vi "Attributes_TCwfm.vi"(2 "data":waveform(dbl)[](array[waveform]), 3 "Refnum in":refnum<k21>) -> (0 "Array":waveform(dbl)[](array[waveform]), 1 "Refnum in 2":refnum<k21>)   [LabVIEW 2017]
uses:
  <resource>/objmgr/daqmx.rc
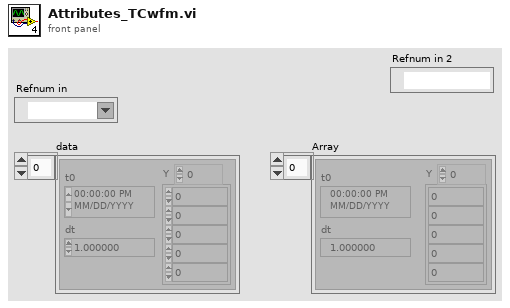
[diagram p1: front panel]
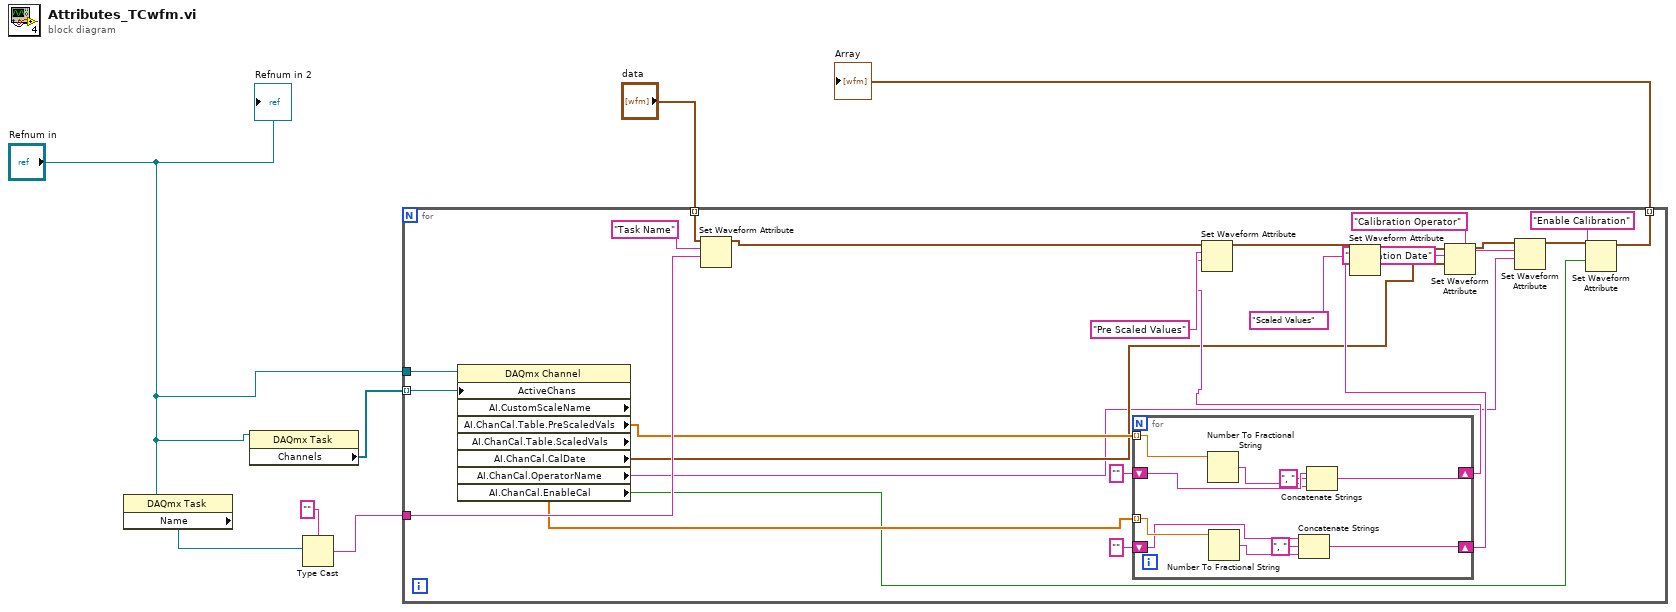
[diagram p0: block diagram]
diagram:
  n1 = property class="DAQmx Task"(reference="Refnum in") -> ("Name"=w4:refnum<k21>)  [unwired: 1 in, 2 out]
  n2 = property class="DAQmx Task"(reference="Refnum in") -> ("Channels"=w1:refnum<k21>[])  [unwired: 1 in, 2 out]
  n3 = Type Cast(type="", x=w4) -> (*(type *) &x=w6:string)
  n4 = for {
    tunnel: "data" -> [w31] mode=indexing
    tunnel: [w8] -> w7 mode=indexing
    tunnel: w6 -> [w30]
    tunnel: "Refnum in" -> [w28]
    tunnel: w1 -> [w27] mode=indexing
    n5 = property class="DAQmx Channel" props=["ActiveChans", "AI.CustomScaleName", "AI.ChanCal.Table.PreScaledVals", "AI.ChanCal.Table.ScaledVals", "AI.ChanCal.CalDate", "AI.ChanCal.OperatorName", "AI.ChanCal.EnableCal"](reference=w28, "ActiveChans"=w27) -> ("AI.ChanCal.Table.PreScaledVals"=w23:dbl[], "AI.ChanCal.Table.ScaledVals"=w22:dbl[], "AI.ChanCal.CalDate"=w16:timestamp, "AI.ChanCal.OperatorName"=w14:string, "AI.ChanCal.EnableCal"=w12:bool)  [unwired: 1 in, 3 out]
    n6 = Set Waveform Attribute(5:w30, 6:"Task Name" ("name"), 7:w31) -> (3:w29:waveform(dbl))  [unwired: 1 in, 2 out]
    n7 = for {
      tunnel: w23 -> [w42] mode=indexing
      tunnel: w22 -> [w39] mode=indexing
      shift-right: [w41] -> w19
      shift-left: "" -> [w40]
      shift-right: [w38] -> w18
      shift-left: "" -> [w37]
      n8 = Number To Fractional String(number=w42) -> (F-format string=w36:string)  [unwired: 3 in]
      n9 = Number To Fractional String(number=w39) -> (F-format string=w34:string)  [unwired: 3 in]
      n10 = Concatenate Strings(w37, ", " ("string"), w34) -> (w38:string)
      n11 = Concatenate Strings(w40, ", " ("string"), w36) -> (w41:string)
    }
    n12 = Set Waveform Attribute(5:w19, 6:"Pre Scaled Values" ("name"), 7:w29) -> (3:w26:waveform(dbl))  [unwired: 1 in, 2 out]
    n13 = Set Waveform Attribute(5:w18, 6:"Scaled Values" ("name"), 7:w26) -> (3:w17:waveform(dbl))  [unwired: 1 in, 2 out]
    n14 = Set Waveform Attribute(5:w16, 6:"Calibration Date" ("name"), 7:w17) -> (3:w10:waveform(dbl))  [unwired: 1 in, 2 out]
    n15 = Set Waveform Attribute(5:w14, 6:"Calibration Operator" ("name"), 7:w10) -> (3:w9:waveform(dbl))  [unwired: 1 in, 2 out]
    n16 = Set Waveform Attribute(5:w12, 6:"Enable Calibration" ("name"), 7:w9) -> (3:w8:waveform(dbl))  [unwired: 1 in, 2 out]
  }
  "Array" <- w7
  "Refnum in 2" <- "Refnum in"
